vi "mcl_disconnect.vi"(8 "error in (no error)":errorcluster, 11 "thorlabs_panel in":refnum<class "mcl_panel.lvclass">) -> (0 "error out":errorcluster, 3 "thorlabs_panel out":refnum<class "mcl_panel.lvclass">)   [LabVIEW 2015, in "mcl_panel.lvclass"]
uses:
  mcl_panel.lvclass
  mcl_piezo_class/mcl_piezo.lvclass
  UI/panel_class/panel.lvclass
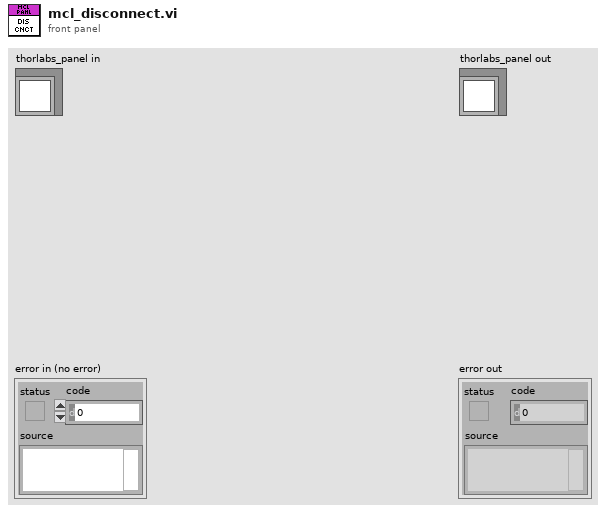
[diagram p1: front panel]
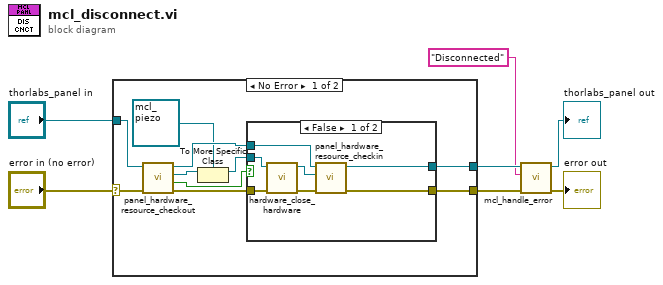
[diagram p0: block diagram]
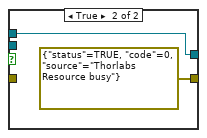
[diagram p2: hidden frame]
diagram:
  n1 = case shown="No Error" "error in (no error)" {
    selector: "error in (no error)" -> [w16 w28]
    tunnel: [w9 w28] -> w4
    tunnel: [w10 w27] -> w5
    tunnel: "thorlabs_panel in" -> [w17 w27]
    frame No Error {
      n2 = call "panel_hardware_resource_checkout.vi"("error in (no error)"=w16, "panel in"=w17) -> ("error out"=w13:errorcluster, "timed out?"=w12:bool, "hardware.lvclass"=w15:refnum<class "hardware.lvclass">, "panel out"=w11:refnum<class "mcl_panel.lvclass">)  [unwired: 6 in]
      n3 = To More Specific Class(target class=refnum<class "mcl_piezo.lvclass"> refnum ("mcl_piezo.lvclass"), reference=w15) -> (specific class reference=w14:refnum<class "mcl_piezo.lvclass">)  [unwired: 1 in, 1 out]
      n4 = case shown="False" w12 {
        tunnel: w14 -> [w20 _]
        tunnel: w13 -> [w21 _]
        tunnel: w11 -> [w22 w25]
        tunnel: [w24 w25] -> w10
        tunnel: [w23 errorcluster {"status"=TRUE, "code"=0, "source"="Thorlabs Resource busy"} ("error out")] -> w9
        frame False {
          n5 = call-dynamic "hardware_close_hardware.vi"("error in (no error)"=w21, "mcl_piezo in"=w20) -> ("error out"=w18:errorcluster, "mcl_piezo out"=w19:refnum<class "mcl_piezo.lvclass">)  [unwired: 8 in]
          n6 = call "panel_hardware_resource_checkin.vi"("error in (no error)"=w18, "hardware.lvclass"=w19, "panel in"=w22) -> ("error out"=w23:errorcluster, "panel out"=w24:refnum<class "mcl_panel.lvclass">)  [unwired: 7 in]
        }
        frame True {
        }
      }
    }
    frame Error {
    }
  }
  n7 = call "mcl_handle_error.vi"("error in (no error)"=w4, "No Error String"="Disconnected", "thorlabs_panel in"=w5) -> ("error out"=→"error out":errorcluster, "thorlabs_panel out"=→"thorlabs_panel out":refnum<class "mcl_panel.lvclass">)  [unwired: 7 in]
